vi "RM-is-moving.vi"(8 "错误输入（无错误）":errorcluster, 11 "MB_Master_Serial输入":refnum<class "MB_Master_Serial.lvclass">) -> (0 "错误输出":errorcluster, 2 "布尔":bool, 3 "MB_Master_Serial输出":refnum<class "MB_Master_Serial.lvclass">)   [LabVIEW 2016]
uses:
  <vilib>/Plasmionique/MB Master/MB Master.lvlib
  <vilib>/Plasmionique/MB Master/MB_Master_Serial/MB_Master_Serial.lvclass
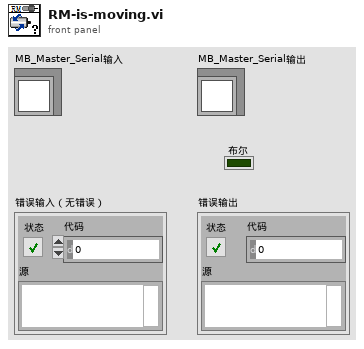
[diagram p1: front panel]
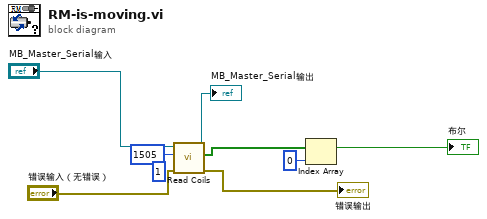
[diagram p0: block diagram]
diagram:
  n1 = call <vilib>:"Read Coils.vi"("error in (no error)"="错误输入（无错误）", "quantity"=u16 1, "starting address"=u16 1505, "MB session in"="MB_Master_Serial输入") -> ("error out"=→"错误输出":errorcluster, "Coils"=w3:bool[], "MB session out"=→"MB_Master_Serial输出":refnum<class "MB_Master_Serial.lvclass">)  [unwired: 5 in]
  n2 = Index Array(array=w3, index=0 ("索引")) -> (element=→"布尔":bool)
